vi "BlinkLight.vi"(11 "Relay In":refnum<visa-resource-name>) -> (3 "Relay Out":refnum<visa-resource-name>)   [LabVIEW 2011]
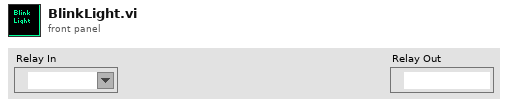
[diagram p1: front panel]
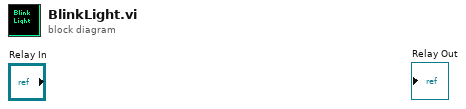
[diagram p0: block diagram]
diagram:
